vi "WSVCAP SHL Host TL RFFE Write Cycle - Multiple DUTs - Common Data.vi"(0 "Data Out (Cycle Commands)":string[](array[string]), 5 "Post Command Delay":dbl[](array[numeric]) format="%#.0p s", 11 "error in":errorcluster, 13 "DUT Mask (All)":bool[](array[boolean])=[TRUE, TRUE, TRUE, TRUE, TRUE, TRUE, TRUE, TRUE, TRUE, TRUE, TRUE, TRUE, TRUE, TRUE, TRUE, TRUE]) -> (15 "error out":errorcluster)   [LabVIEW 2012]
panel:
  out "Socket Mask":u16=1 format="%02x"
  out "RFFE Data Out [U8]":u8[][](array[numeric]) format="%02x"
  # "DUT 01"
  # "DUT 02"
  # "DUT 03"
  # "DUT 04"
  # "DUT 05"
  # "DUT 06"
  # "DUT 07"
  # "DUT 08"
  # "DUT 09"
  # "DUT 10"
  # "DUT 11"
  # "DUT 12"
  # "DUT 13"
  # "DUT 14"
  # "DUT 15"
  # "DUT 16"
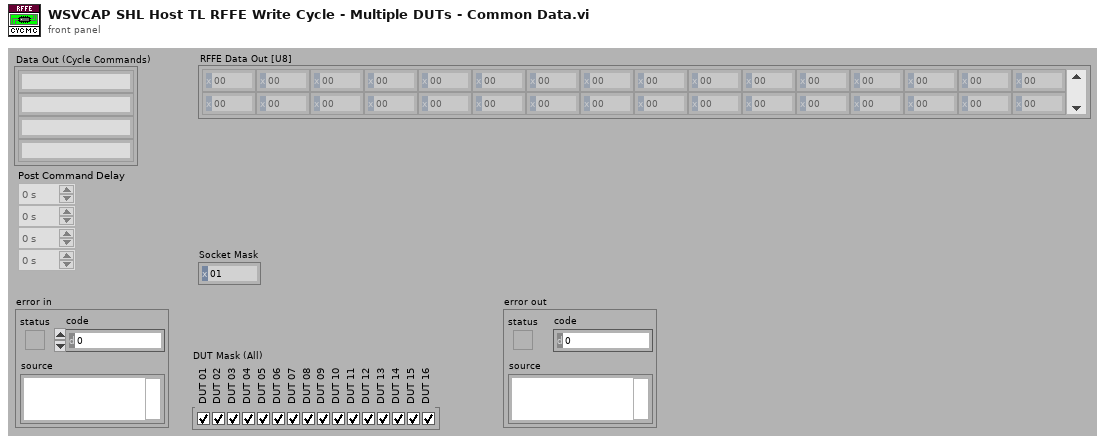
[diagram p1: front panel]
types:
  T1 = typedef "WSVCAP SHL Core System Cluster.ctl" = cluster{"Settings":T2, "FPGA Resource":tag, "Online":bool, "I2C Wait Ticks":u32, "SPI Wait Ticks":u32, "RFFE Wait Ticks":u32}
  T2 = typedef "WSVCAP SHL I2C Settings Cluster.ctl" = cluster{"FPGA Resource Name":string, "I2C Slave Address":u8, "I2C Clock Rate (Hz)":dbl, "SPI Clock Rate (Hz)":dbl, "RFFE Slave Address":u8, "RFFE Clock Rate (Hz)":dbl, "Simulate FPGA":bool, "C1 Cap DAC Default":u8, "C2 Cap DAC Default":u8, "C3 Cap DAC Default":u8}
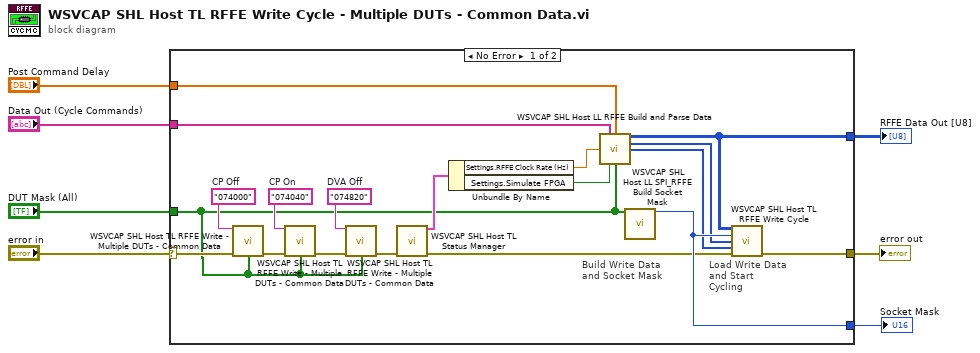
[diagram p0: block diagram]
diagram:
  n1 = case shown="No Error" "error in" {
    selector: "error in" -> [w14 _]
    tunnel: [w26 _] -> w7
    tunnel: [w25 _] -> w5
    tunnel: [w24 _] -> w4
    tunnel: "DUT Mask (All)" -> [w8 _]
    tunnel: "Post Command Delay" -> [w23 _]
    tunnel: "Data Out (Cycle Commands)" -> [w22 _]
    frame No Error {
      w9 = "074820"  # DVA Off
      w10 = "074040"  # CP On
      w11 = "074000"  # CP Off
      # "Load Write Data and Start Cycling"
      # "Build Write Data and Socket Mask"
      n2 = call "WSVCAP SHL Host TL RFFE Write - Multiple DUTs - Common Data.vi"("Data Out"=w11, "error in"=w14, "DUT Mask (All)"=w8) -> ("error out"=w15:errorcluster)  [unwired: 12 in]
      n3 = call "WSVCAP SHL Host TL RFFE Write - Multiple DUTs - Common Data.vi"("Data Out"=w10, "error in"=w15, "DUT Mask (All)"=w8) -> ("error out"=w13:errorcluster)  [unwired: 12 in]
      n4 = call "WSVCAP SHL Host TL RFFE Write - Multiple DUTs - Common Data.vi"("Data Out"=w9, "error in"=w13, "DUT Mask (All)"=w8) -> ("error out"=w12:errorcluster)  [unwired: 12 in]
      n5 = call "WSVCAP SHL Host TL Status Manager.vi"("error in"=w12) -> ("System Out"=w21:T1, "error out"=w20:errorcluster)  [unwired: 13 in]
      n6 = Unbundle By Name(w21) -> ("Settings.RFFE Clock Rate (Hz)"=w16:dbl, "Settings.Simulate FPGA"=w19:bool)
      n7 = call "WSVCAP SHL Host LL RFFE Build and Parse Data.vi"("Data Out (Cycle Commands)"=w22, "Post Command Delay"=w23, "Clock Rate (Hz) (Cycle Only)"=w16, "Simulate FPGA (Cycle Only)"=w19, "DUT Mask (All)"=w8) -> ("RFFE Data Out [U8]"=w25:u8[][], "CMD Lengths (Bits)"=w18:u8[], "CMD Delays (Ticks)"=w17:u32[])  [unwired: 7 in, 1 out]
      n8 = call "WSVCAP SHL Host LL SPI_RFFE Build Socket Mask.vi"("DUT Mask"=w8) -> ("Socket Mask [U16]"=w24:u16)  [unwired: 13 in, 1 out]
      n9 = call "WSVCAP SHL Host TL RFFE Write Cycle.vi"("RFFE Data Out"=w25, "Socket Mask"=w24, "Cycle CMD Lengths (bits)"=w18, "Cycle CMD Delay (ticks)"=w17, "error in"=w20) -> ("error out"=w26:errorcluster)  [unwired: 10 in]
    }
    frame Error {
    }
  }
  "error out" <- w7
  "RFFE Data Out [U8]" <- w5
  "Socket Mask" <- w4
